vi "createXLS.vi"(8 "error in (no error)":errorcluster, 11 "MS-Excel in":refnum<class "MS-Excel.lvclass">) -> (0 "error out":errorcluster, 3 "MS-Excel out":refnum<class "MS-Excel.lvclass">)   [LabVIEW 2017, in "LabVIEW NPOI.lvlib" / "MS-Excel.lvclass"]
uses:
  MS-Excel.lvclass
  C:/Users/Neo/Desktop/Dev_Tools_BR/LabVIEW_NPOI/src/LabVIEW NPOI/Document/Document.lvclass
  Document/Document.lvclass/Document.ctl
  C:/Users/Neo/Desktop/Dev_Tools_BR/LabVIEW_NPOI/src/lib/NPOI 2.1.1/NPOI.dll
  lib/NPOI 2.1.1/NPOI.dll
  Document/Get FilePath.vi
  Support/File Stream/File Stream.lvlib
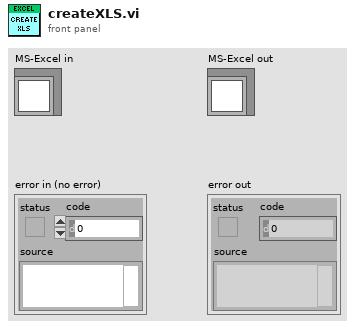
[diagram p1: front panel]
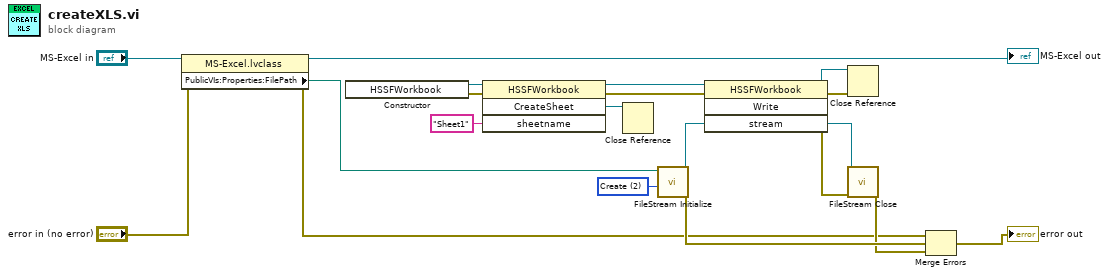
[diagram p0: block diagram]
diagram:
  w1 = 2 items=["CreateNew"=1, "Create"=2, "Open"=3, "OpenOrCreate"=4, "Truncate"=5, "Append"=6] ("mode")
  n1 = property class="MS-Excel.lvclass"(reference="MS-Excel in", error in="error in (no error)") -> (reference out=→"MS-Excel out":refnum<class "MS-Excel.lvclass">, error out=w8:errorcluster, "PublicVIs:Properties:FilePath"=w12:path)
  n2 = constructor class="HSSFWorkbook"() -> (reference out=w17:refnum<k24>, error out=w18:errorcluster)  [unwired: 3 in, 1 out]
  n3 = invoke class="HSSFWorkbook" method="CreateSheet"(reference=w17, error in=w18, "sheetname"="Sheet1") -> (reference out=w15:refnum<k24>, error out=w13:errorcluster, "CreateSheet"=w11:refnum<k24>)  [unwired: 1 in, 1 out]
  n4 = Close Reference(reference=w11) -> ()  [unwired: 1 in, 1 out]
  n5 = call "FileStream Initialize.vi"("mode"=w1, "path"=w12) -> ("error out"=w10:errorcluster, "new reference"=w14:refnum<k24>)  [unwired: 8 in]
  n6 = invoke class="HSSFWorkbook" method="Write"(reference=w15, error in=w13, "stream"=w14) -> (reference out=w3:refnum<k24>, error out=w2:errorcluster)  [unwired: 1 in, 2 out]
  n7 = Close Reference(reference=w3, error in (no error)=w2) -> ()  [unwired: 1 out]
  n8 = call "FileStream Close.vi"("error in (no error)"=w2, "reference"=w14) -> ("error out"=w9:errorcluster)  [unwired: 9 in]
  n9 = Merge Errors(w8, w10, w9) -> (→"error out":errorcluster)
